vi "Enable Video UI.vi"(8 "error in (no error)":errorcluster, 11 "SB App in":refnum<class "SB App.lvclass">) -> (0 "error out":errorcluster, 3 "SB App out":refnum<class "SB App.lvclass">)   [LabVIEW 2020, in "SB App.lvlib" / "SB App.lvclass"]
uses:
  SB App.lvclass
  Video Prefs.ctl
  561f683e-207c-49c0-870c-3556ed295013.vi
  02dc37d3-337f-40b0-987c-e8995710b534.vi
  Prefs INI Path.vi
  <vilib>/Utility/sysdir.llb/Get System Directory.vi
  <vilib>/Utility/config.llb/Open Config Data.vi
  <vilib>/Utility/config.llb/Read Key.vi
  <vilib>/Utility/config.llb/Read Key (Path).vi
  <vilib>/Utility/config.llb/Close Config Data.vi
  <vilib>/Utility/config.llb/Read Key (String).vi
panel:
  in  "Filename Format":string
  in  "Cancel Button":bool
  in  "OK Button":bool
  in  "Folder to Save Videos":path
  # "Configure Video saving options:"
  # "MP4 files will be created using this name. \".mp4\" is always added to the end. Options include:\n\n<Teams> - Team names separated by Hyphens\n<Time> - Timestamp of video creation at the end of the match\n\nAny other text will left as-is."
  # "Configured options are saved to Prefs and will be used again when re-enabling video saving."
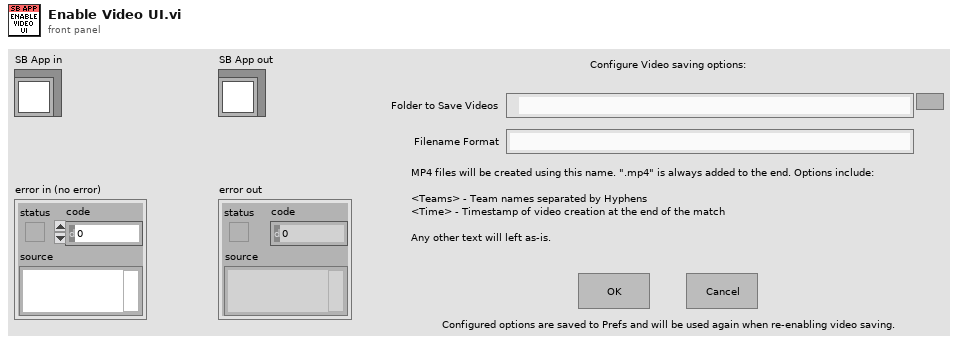
[diagram p1: front panel]
types:
  T1 = enum32{"Invalid", "Standard", "Closed", "Hidden", "Minimized", "Maximized"}
  T2 = typedef "SB App.lvlib/SB App.lvclass/Video Prefs.ctl" = cluster{"Video Enabled":bool, "Video Path":path, "Filename Format":string}
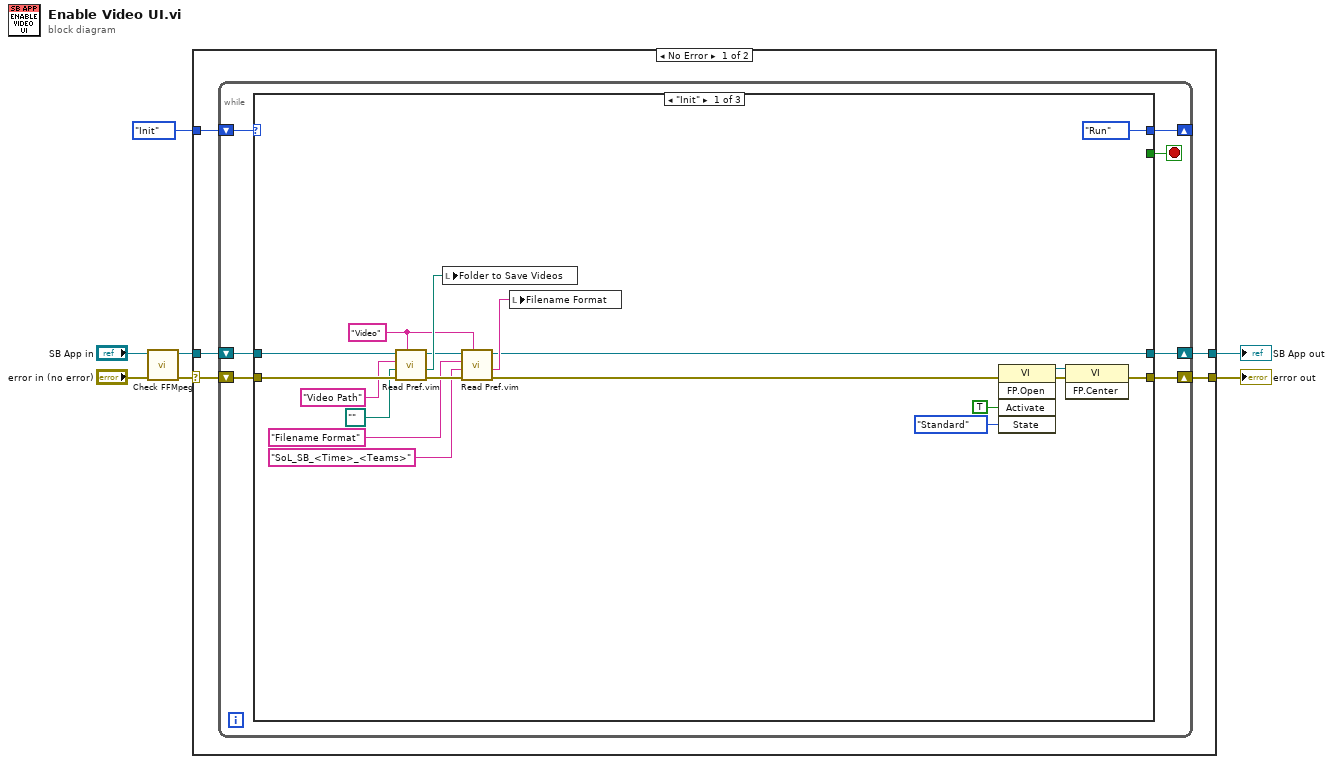
[diagram p0: block diagram]
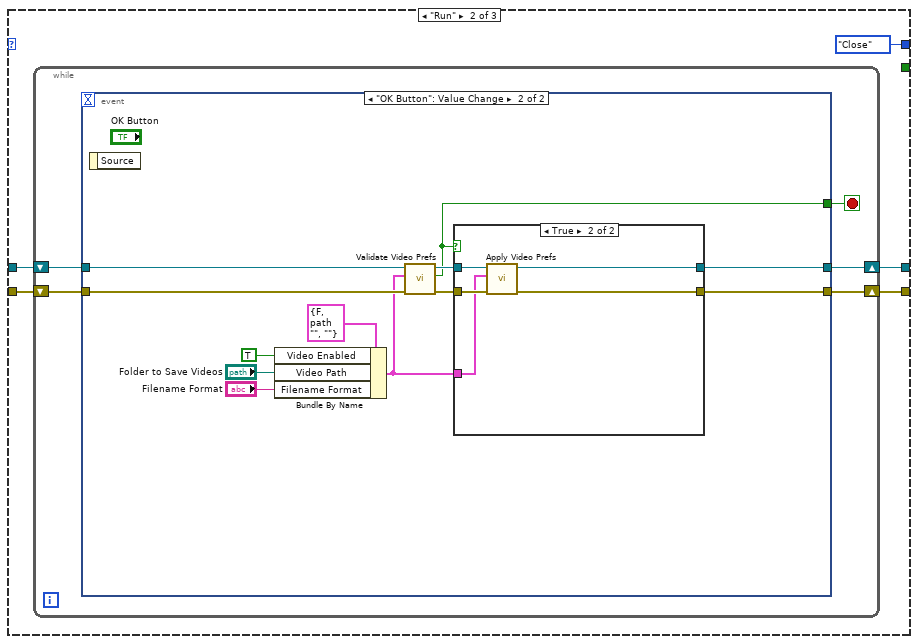
[diagram p2: hidden frame]
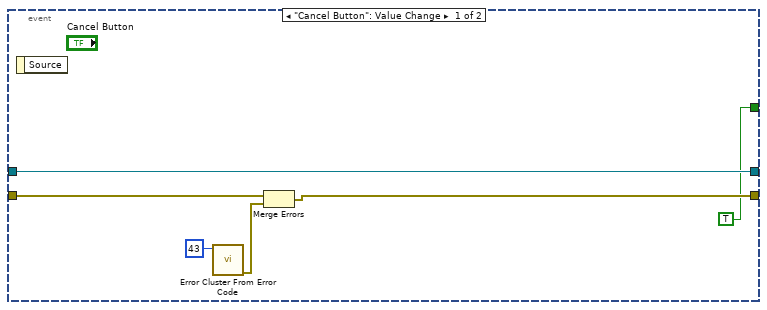
[diagram p3: hidden frame]
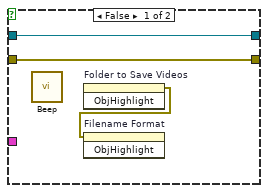
[diagram p4: hidden frame]
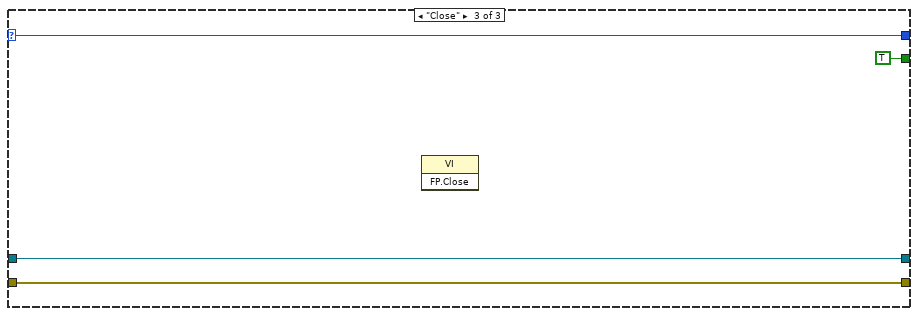
[diagram p5: hidden frame]
diagram:
  n1 = call "Check FFMpeg.vi"("error in (no error)"="error in (no error)", "SB App in"="SB App in") -> ("error out"=w5:errorcluster, "SB App out"=w4:refnum<class "SB App.lvclass">)  [unwired: 8 in]
  n2 = case shown="No Error" w5 {
    selector: w5 -> [w11 w79]
    tunnel: w4 -> [w12 w80]
    tunnel: [w10 w80] -> w3
    tunnel: [w9 w79] -> w2
    tunnel: enum16{"Init", "Run", "Close"}."Init" ("Basic UI State") -> [w8 _]
    frame No Error {
      n3 = while {
        shift-right: [w13] -> w10
        shift-left: w12 -> [w18]
        shift-right: [w14] -> w9
        shift-left: w11 -> [w17]
        shift-right: [w16] -> _
        shift-left: w8 -> [w19]
        stop <- w15 stop-if-true
        n4 = case shown="\"Init\"" w19 {
          selector: w19 -> [_ _ w78]
          tunnel: w18 -> [w32 w42 w76]
          tunnel: w17 -> [w31 w41 w75]
          tunnel: [enum16{"Init", "Run", "Close"}."Run" ("Basic UI State") enum16{"Init", "Run", "Close"}."Close" ("Basic UI State") w78] -> w16
          tunnel: [_ _ TRUE] -> w15
          tunnel: [w33 w39 w75] -> w14
          tunnel: [w21 w40 w76] -> w13
          frame "Init" {
            w25 = "Video" ("Section")
            n5 = call "Read Pref.vim"("Section"=w25, "error in (no error)"=w31, "Type / Default (String)"=path "", "Key"="Video Path", "SB App in"=w32) -> ("error out"=w26:errorcluster, "value"=w28:path, "SB App out"=w27:refnum<class "SB App.lvclass">)  [unwired: 3 in, 1 out]
            n6 = local write "Folder to Save Videos"(w28) -> ()
            n7 = call "Read Pref.vim"("Section"=w25, "error in (no error)"=w26, "Type / Default (String)"="SoL_SB_<Time>_<Teams>" ("Key"), "Key"="Filename Format", "SB App in"=w27) -> ("error out"=w20:errorcluster, "value"=w22:string, "SB App out"=w21:refnum<class "SB App.lvclass">)  [unwired: 3 in, 1 out]
            n8 = local write "Filename Format"(w22) -> ()
            n9 = invoke class="VI" method="FP.Open"(error in=w20, "Activate"=TRUE ("Activate?"), "State"=T1."Standard") -> (reference out=w35:refnum<vi>, error out=w34:errorcluster)  [unwired: 2 in, 3 out]
            n10 = invoke class="VI" method="FP.Center"(reference=w35, error in=w34) -> (error out=w33:errorcluster)  [unwired: 1 in, 2 out]
          }
          frame "Run" {
            n11 = while {
              shift-right: [w46] -> w40
              shift-left: w42 -> [w48]
              shift-right: [w45] -> w39
              shift-left: w41 -> [w47]
              stop <- w44 stop-if-true
              n12 = event shown="[1] \"OK Button\": Value Change" {
                selector: _ -> [_ _]
                dyn-events: _ -> [_ _]
                timeout: _ -> [_ _]
                tunnel: w48 -> [w54 w62]
                tunnel: w47 -> [w52 w61]
                tunnel: [w54 w57] -> w46
                tunnel: [w50 w56] -> w45
                tunnel: [TRUE w55] -> w44
                event "Cancel Button": Value Change {
                  n13 = event-data() -> ()  [unwired: 1 in, 1 out]
                  n14 = call <vilib>:"Error Cluster From Error Code.vi"("error code (0)"=43) -> ("error out"=w51:errorcluster)  [unwired: 8 in]
                  n15 = Merge Errors(w52, w51) -> (w50:errorcluster)
                }
                event "OK Button": Value Change {
                  n16 = event-data() -> ()  [unwired: 1 in, 1 out]
                  n17 = Bundle By Name(cluster=T2 {"Video Enabled"=FALSE, "Video Path"=path "", "Filename Format"=""} ("Video Prefs"), "Video Enabled"=TRUE, "Video Path"="Folder to Save Videos", "Filename Format"="Filename Format") -> (w58:T2)
                  n18 = call "Validate Video Prefs.vi"("error in (no error)"=w61, "Video Prefs"=w58, "SB App in"=w62) -> ("error out"=w59:errorcluster, "Valid?"=w55:bool, "SB App out"=w60:refnum<class "SB App.lvclass">)  [unwired: 6 in]
                  n19 = case shown="True" w55 {
                    tunnel: w60 -> [w69 w74]
                    tunnel: w59 -> [w68 w73]
                    tunnel: w58 -> [_ w72]
                    tunnel: [w69 w71] -> w57
                    tunnel: [w68 w70] -> w56
                    frame False {
                      n20 = call <vilib>:"Beep.vi"() -> ()  [unwired: 12 in]
                      n21 = invoke on="Folder to Save Videos" class="Path" method="ObjHighlight"() -> (error out=w67:errorcluster)  [unwired: 3 in, 2 out]
                      n22 = invoke on="Filename Format" class="Str" method="ObjHighlight"(error in=w67) -> ()  [unwired: 2 in, 3 out]
                    }
                    frame True {
                      n23 = call "Apply Video Prefs.vi"("error in (no error)"=w73, "Video Prefs"=w72, "SB App in"=w74) -> ("error out"=w70:errorcluster, "SB App out"=w71:refnum<class "SB App.lvclass">)  [unwired: 7 in]
                    }
                  }
                }
              }
            }
          }
          frame "Close" {
            n24 = invoke class="VI" method="FP.Close"() -> ()  [unwired: 3 in, 3 out]
          }
        }
      }
    }
    frame Error {
    }
  }
  "error out" <- w2
  "SB App out" <- w3
